vi "Case structures 1.vi"() -> ()   [LabVIEW 2022 SP3]
panel:
  out "Numeric":dbl
  in  "y":dbl
  in  "x":dbl
  in  "Boolean":bool
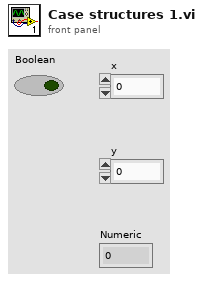
[diagram p1: front panel]
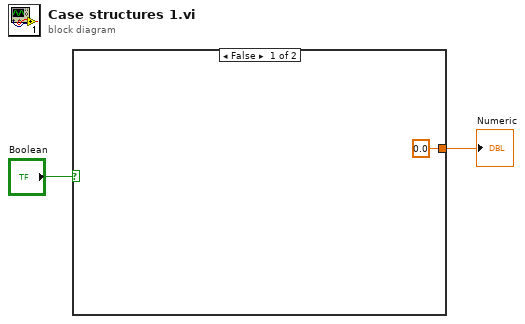
[diagram p0: block diagram]
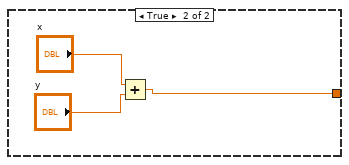
[diagram p2: hidden frame]
diagram:
  n1 = case shown="False" "Boolean" {
    tunnel: [0.0 w4] -> w1
    frame False {
    }
    frame True {
      n2 = Add(x="x", y="y") -> (x+y=w4:dbl)
    }
  }
  "Numeric" <- w1
